vi "Customize Menu.vi"(6 "Display information":T1, 8 "error in":errorcluster, 11 "menu reference":refnum<k9>) -> (0 "error out":errorcluster)   [LabVIEW 2014]
uses:
  <vilib>/Utility/miscctls.llb/LVMenuShortCut.ctl
  Data Logger Global Variable.vi
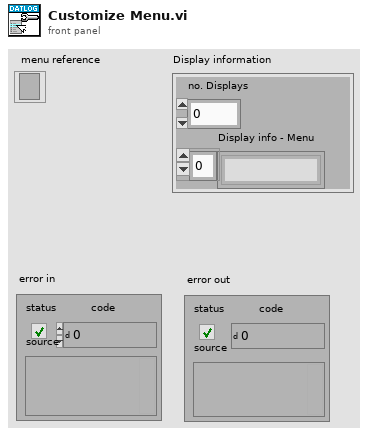
[diagram p1: front panel]
types:
  T1 = cluster{"no. Displays":i32, "Display info - Menu":string[]}
  T2 = typedef "LVMenuShortCut.ctl" = cluster{"Include Shift Key?":bool, "Include Ctrl Key?":bool, "Shortcut Key":string}
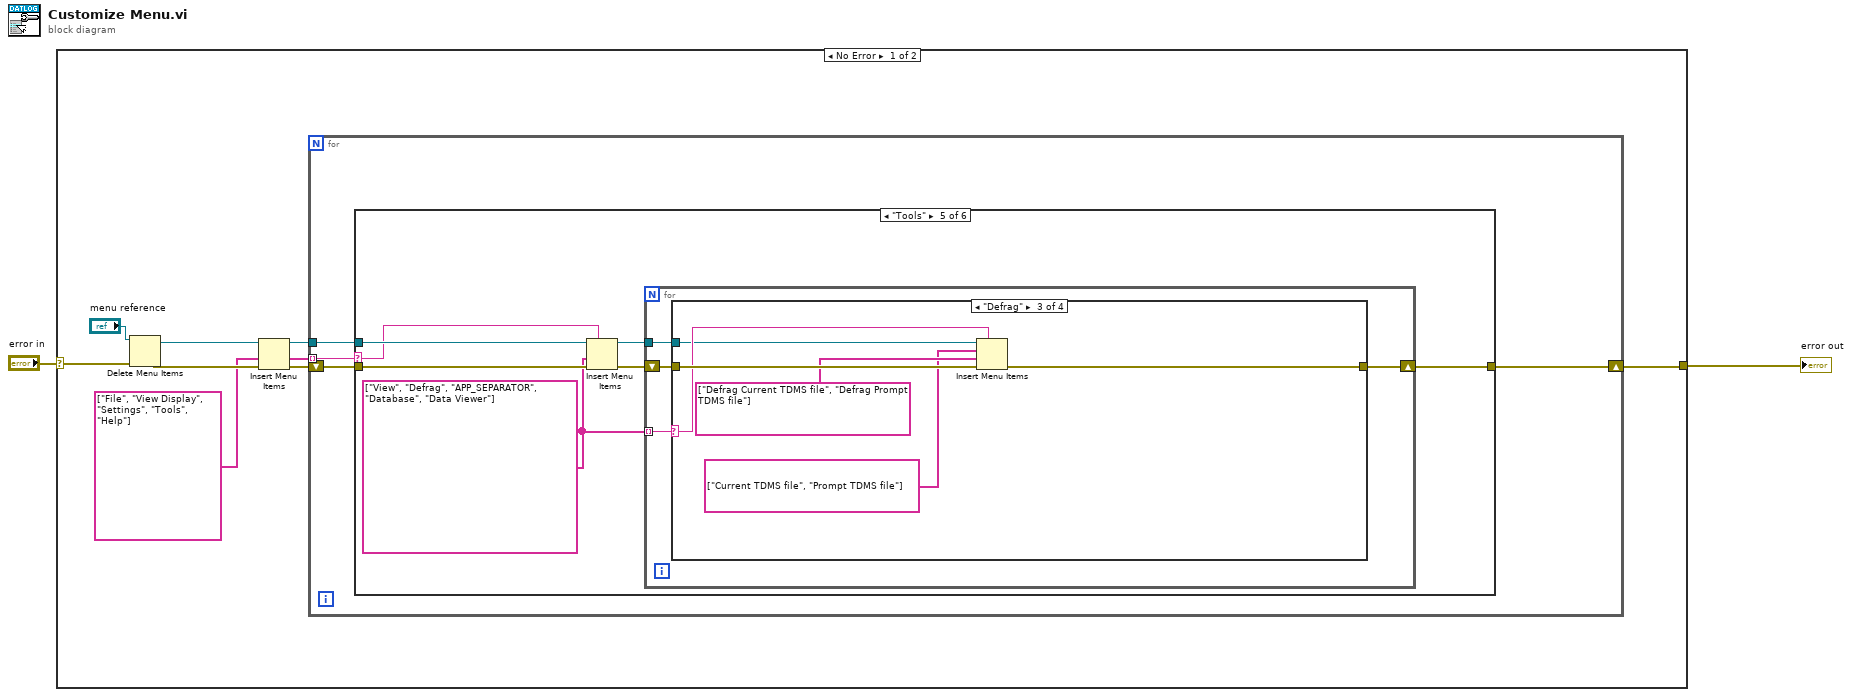
[diagram p0: block diagram]
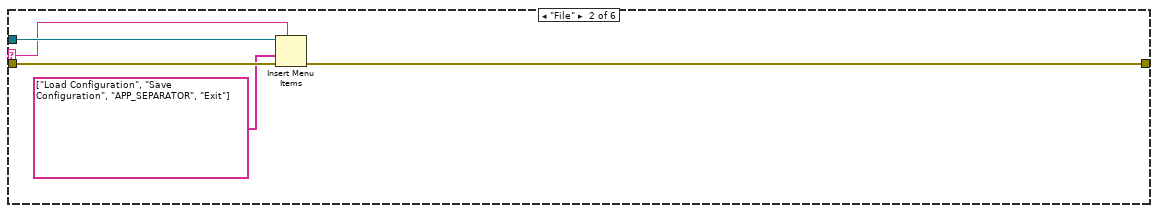
[diagram p3: hidden frame]
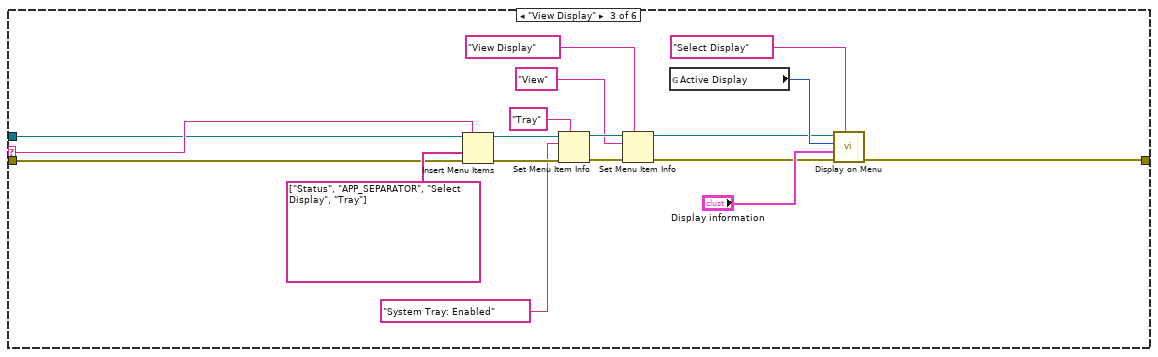
[diagram p4: hidden frame]
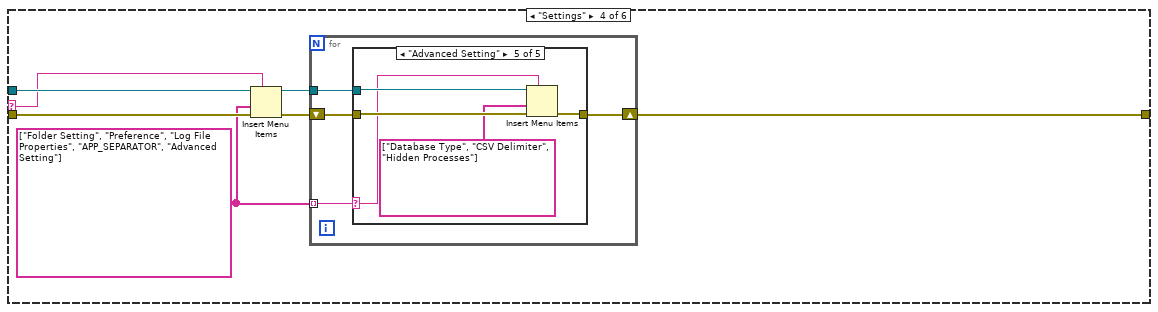
[diagram p5: hidden frame]
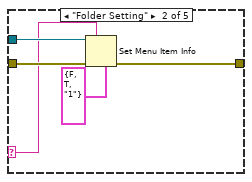
[diagram p7: hidden frame]
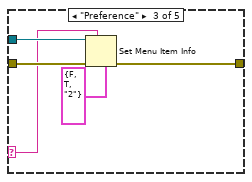
[diagram p8: hidden frame]
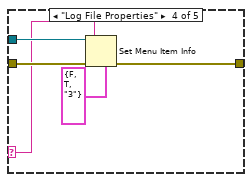
[diagram p9: hidden frame]
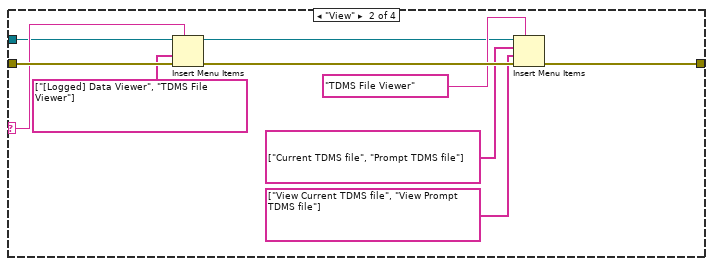
[diagram p11: hidden frame]
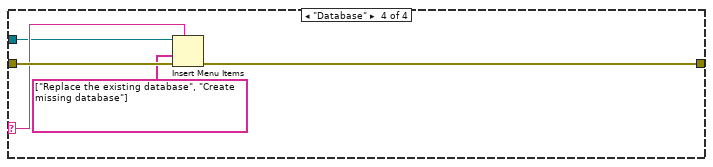
[diagram p12: hidden frame]
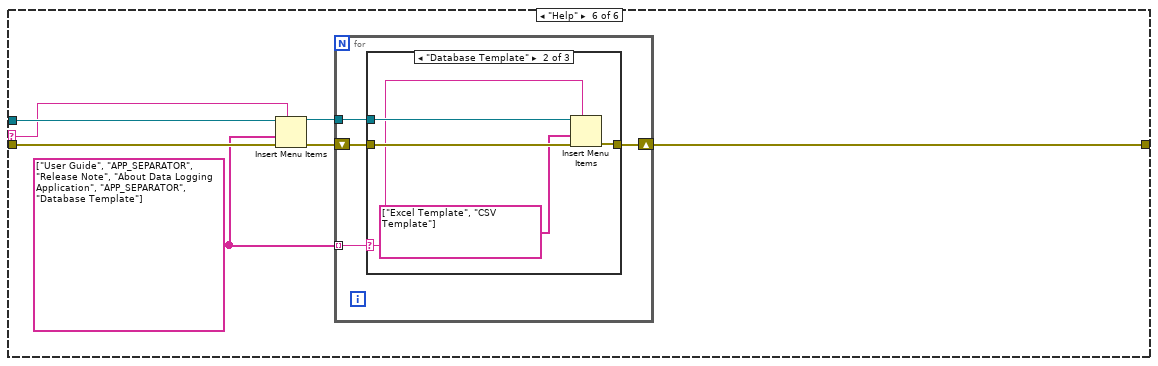
[diagram p13: hidden frame]
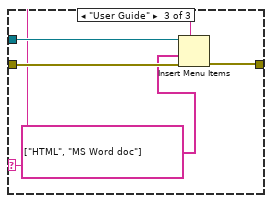
[diagram p15: hidden frame]
diagram:
  n1 = case shown="No Error" "error in" {
    selector: "error in" -> [w10 w127]
    tunnel: [w3 w127] -> w1
    frame No Error {
      n2 = Delete Menu Items(6:w10, 9:"menu reference") -> (0:w9:errorcluster, 3:w8:refnum<k9>)  [unwired: 2 in]
      n3 = Insert Menu Items(6:w9, 7:string[] ["File", "View Display", "Settings", "Tools", "Help"] ("item tags"), 9:w8) -> (0:w5:errorcluster, 1:w4:string[], 3:w6:refnum<k9>)  [unwired: 3 in]
      n4 = for {
        tunnel: w6 -> [w15]
        shift-right: [w13] -> w3
        shift-left: w5 -> [w12]
        tunnel: w4 -> [w14] mode=indexing
        n5 = case shown="\"Tools\"" w14 {
          selector: w14 -> [_ w19 w31 w44 w76 w109]
          tunnel: w15 -> [_ w21 w30 w46 w78 w111]
          tunnel: [w16 w18 w32 w41 w74 w107] -> w13
          tunnel: w12 -> [w16 w20 w33 w45 w77 w110]
          frame "do nothing", Default {
          }
          frame "File" {
            n6 = Insert Menu Items(5:w19, 6:w20, 7:string[] ["Load Configuration", "Save Configuration", "APP_SEPARATOR", "Exit"] ("item tags"), 9:w21) -> (0:w18:errorcluster)  [unwired: 2 in, 2 out]
          }
          frame "View Display" {
            n7 = Insert Menu Items(5:w31, 6:w33, 7:string[] ["Status", "APP_SEPARATOR", "Select Display", "Tray"] ("item tags"), 9:w30) -> (0:w37:errorcluster, 3:w36:refnum<k9>)  [unwired: 2 in, 1 out]
            n8 = Set Menu Item Info(7:"Tray", 8:w37, 10:"System Tray: Enabled", 11:w36) -> (0:w26:errorcluster, 3:w27:refnum<k9>)  [unwired: 3 in]
            n9 = Set Menu Item Info(7:"View Display", 8:w26, 10:"View", 11:w27) -> (0:w24:errorcluster, 3:w25:refnum<k9>)  [unwired: 3 in]
            n10 = global read "Data Logger Global Variable.vi" "Active Display"() -> (w28:u16)
            n11 = call "Display on Menu.vi"("Menu Tag"="Select Display", "error in"=w24, "Display information"="Display information", "Active Display"=w28, "Menu Ref"=w25) -> ("error out"=w32:errorcluster)  [unwired: 5 in, 1 out]
          }
          frame "Settings" {
            w40 = string[] ["Folder Setting", "Preference", "Log File Properties", "APP_SEPARATOR", "Advanced Setting"] ("item tags")
            n12 = Insert Menu Items(5:w44, 6:w45, 7:w40, 9:w46) -> (0:w43:errorcluster, 3:w42:refnum<k9>)  [unwired: 2 in, 1 out]
            n13 = for {
              shift-right: [w48] -> w41
              shift-left: w43 -> [w49]
              tunnel: w42 -> [w50]
              tunnel: w40 -> [w47] mode=indexing
              n14 = case shown="\"Advanced Setting\"" w47 {
                selector: w47 -> [_ w52 w57 w62 w68]
                tunnel: w50 -> [_ w56 w61 w66 w69]
                tunnel: w49 -> [w51 w55 w60 w65 w70]
                tunnel: [w51 w54 w59 w64 w71] -> w48
                frame "False", Default {
                }
                frame "Folder Setting" {
                  n15 = Set Menu Item Info(4:T2 {"Include Shift Key?"=FALSE, "Include Ctrl Key?"=TRUE, "Shortcut Key"="1"} ("short cut"), 7:w52, 8:w55, 11:w56) -> (0:w54:errorcluster)  [unwired: 3 in, 1 out]
                }
                frame "Preference" {
                  n16 = Set Menu Item Info(4:T2 {"Include Shift Key?"=FALSE, "Include Ctrl Key?"=TRUE, "Shortcut Key"="2"} ("short cut"), 7:w57, 8:w60, 11:w61) -> (0:w59:errorcluster)  [unwired: 3 in, 1 out]
                }
                frame "Log File Properties" {
                  n17 = Set Menu Item Info(4:T2 {"Include Shift Key?"=FALSE, "Include Ctrl Key?"=TRUE, "Shortcut Key"="3"} ("short cut"), 7:w62, 8:w65, 11:w66) -> (0:w64:errorcluster)  [unwired: 3 in, 1 out]
                }
                frame "Advanced Setting" {
                  n18 = Insert Menu Items(5:w68, 6:w70, 7:string[] ["Database Type", "CSV Delimiter", "Hidden Processes"] ("item tags"), 9:w69) -> (0:w71:errorcluster)  [unwired: 2 in, 2 out]
                }
              }
            }
          }
          frame "Tools" {
            w73 = string[] ["View", "Defrag", "APP_SEPARATOR", "Database", "Data Viewer"] ("item tags")
            n19 = Insert Menu Items(5:w76, 6:w77, 7:w73, 9:w78) -> (0:w75:errorcluster, 3:w72:refnum<k9>)  [unwired: 2 in, 1 out]
            n20 = for {
              shift-right: [w81] -> w74
              shift-left: w75 -> [w82]
              tunnel: w73 -> [w80] mode=indexing
              tunnel: w72 -> [w79]
              n21 = case shown="\"Defrag\"" w80 {
                selector: w80 -> [_ w91 w96 w101]
                tunnel: w82 -> [w83 w93 w99 w104]
                tunnel: [w83 w88 w98 w103] -> w81
                tunnel: w79 -> [_ w90 w95 w100]
                frame "do nothing", Default {
                }
                frame "View" {
                  n22 = Insert Menu Items(5:w91, 6:w93, 7:string[] ["[Logged] Data Viewer", "TDMS File Viewer"] ("item tags"), 9:w90) -> (0:w89:errorcluster, 3:w86:refnum<k9>)  [unwired: 2 in, 1 out]
                  n23 = Insert Menu Items(5:"TDMS File Viewer", 6:w89, 7:string[] ["View Current TDMS file", "View Prompt TDMS file"] ("item tags"), 8:string[] ["Current TDMS file", "Prompt TDMS file"] ("item tags"), 9:w86) -> (0:w88:errorcluster)  [unwired: 1 in, 2 out]
                }
                frame "Defrag" {
                  n24 = Insert Menu Items(5:w96, 6:w99, 7:string[] ["Defrag Current TDMS file", "Defrag Prompt TDMS file"] ("item tags"), 8:string[] ["Current TDMS file", "Prompt TDMS file"] ("item tags"), 9:w95) -> (0:w98:errorcluster)  [unwired: 1 in, 2 out]
                }
                frame "Database" {
                  n25 = Insert Menu Items(5:w101, 6:w104, 7:string[] ["Replace the existing database", "Create missing database"] ("item tags"), 9:w100) -> (0:w103:errorcluster)  [unwired: 2 in, 2 out]
                }
              }
            }
          }
          frame "Help" {
            w106 = string[] ["User Guide", "APP_SEPARATOR", "Release Note", "About Data Logging Application", "APP_SEPARATOR", "Database Template"] ("item tags")
            n26 = Insert Menu Items(5:w109, 6:w110, 7:w106, 9:w111) -> (0:w108:errorcluster, 3:w105:refnum<k9>)  [unwired: 2 in, 1 out]
            n27 = for {
              shift-right: [w113] -> w107
              shift-left: w108 -> [w114]
              tunnel: w106 -> [w115] mode=indexing
              tunnel: w105 -> [w112]
              n28 = case shown="\"Database Template\"" w115 {
                selector: w115 -> [_ w118 w123]
                tunnel: w114 -> [w116 w121 w126]
                tunnel: [w116 w120 w125] -> w113
                tunnel: w112 -> [_ w119 w124]
                frame "False", Default {
                }
                frame "Database Template" {
                  n29 = Insert Menu Items(5:w118, 6:w121, 7:string[] ["Excel Template", "CSV Template"] ("item tags"), 9:w119) -> (0:w120:errorcluster)  [unwired: 2 in, 2 out]
                }
                frame "User Guide" {
                  n30 = Insert Menu Items(5:w123, 6:w126, 7:string[] ["HTML", "MS Word doc"] ("item tags"), 9:w124) -> (0:w125:errorcluster)  [unwired: 2 in, 2 out]
                }
              }
            }
          }
        }
      }
    }
    frame Error {
    }
  }
  "error out" <- w1
